vi "FTW-MessagePayload-Compose.vi"(2 "Message Body":string, 3 "Message Header":string, 4 "Sender Identity":string) -> (0 "Message":T1)   [LabVIEW 2015]
uses:
  FTW-MessagePayload.ctl
panel:
  # "Inputs"
  # "Outputs"
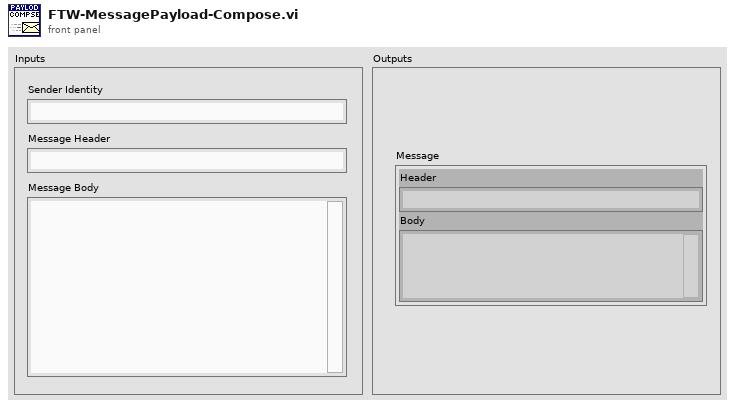
[diagram p1: front panel]
types:
  T1 = typedef "FTW-MessagePayload.ctl" = cluster{"Header":string, "Body":string, "FTW: Sender Identity":string, "FTW: Reply Address":string, "FTW: Reply Error":errorcluster}
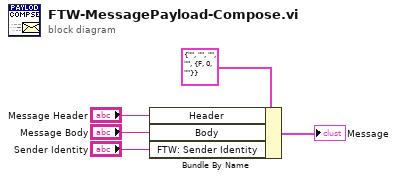
[diagram p0: block diagram]
diagram:
  n1 = Bundle By Name(cluster=T1 {"Header"="", "Body"="", "FTW: Sender Identity"="", "FTW: Reply Address"="", "FTW: Reply Error"={"status"=FALSE, "code"=0, "source"=""}} ("Message"), "Header"="Message Header", "Body"="Message Body", "FTW: Sender Identity"="Sender Identity") -> (→"Message":T1)
